vi "VISA_Simple Serial.vi"(0 "VISA resource name":refnum<visa-resource-name>="COM1", 5 "Command":string="*IDN?\\n", 7 "delay before read (ms)":u32=500, 9 "Serial Settings":T1={"baud rate"=9600, "data bits"=8, "parity"=enum."None", "stop bits"=10, "flow control"=0} {"flow control" items=["None"=0, "XON/XOFF"=1, "RTS/CTS"=2, "DTR/DSR"=4]; "stop bits" items=["1.0"=10, "1.5"=15, "2.0"=20]; "data bits" min=5 max=8 step=1; "baud rate" items=["75"=75, "110"=110, "134"=134, "150"=150, "300"=300, "600"=600, "1200"=1200, "1800"=1800, "2400"=2400, "4800"=4800, "7200"=7200, "9600"=9600, "14400"=14400, "19200"=19200, "28800"=28800, "38400"=38400, "56000"=56000, "57600"=57600, "115200"=115200, "128000"=128000, "230400"=230400]}, 11 "error in (no error)":errorcluster) -> (4 "Response":string, 6 "bytes read":u32, 15 "error out":errorcluster)   [LabVIEW 2021, in "Communication.lvlib"]
doc: "<B>Note: This VI is taken from LabVIEW example located at C:\\Program Files (x86)\\National Instruments\\LabVIEW <version>\\examples\\Instrument IO\\Serial\\Simple Serial.vi. More such examples can be found in the same location.</B>\n\nThis example performs a serial port write and a serial port read. The parameters set for the serial port must match the parameters of the connected instrument or device. The VISA Configure Serial Port VI sets the configuration parameters. The front panel displays the controls used to configure the basic parameters, such as baud rate, data bits, and parity. The VI passes the VISA resource name to other VIs that perform operations on that VISA resource. The VISA Write function sends a command to the serial device and the VISA Read function returns data based on the command. The VISA Close function then closes the reference to the serial device. It is important to close the reference; otherwise, further communication through that port might not be possible."
uses:
  Communication.lvlib
  Typedefs/Serial - Settings.ctl
  <vilib>/Instr/_visa.llb/VISA Configure Serial Port (Instr).vi
panel:
  # "Overview: Demonstrates the use of the VISA functions to send a single command to a serial instrument and read a response.\nRequirements: NI-VISA Driver\nInstructions:\n1. Ensure the resource specified by the VISA resource name is a valid serial device.\n2. Enter the serial visa command / query.\n3. Update other configuration required to establish serial communication.\n4. Run the VI."
  # "Note: This VI is taken from LabVIEW example located at C:\\Program Files (x86)\\National Instruments\\LabVIEW <version>\\examples\\Instrument IO\\Serial\\Simple Serial.vi.  More such examples can be found in the same location."
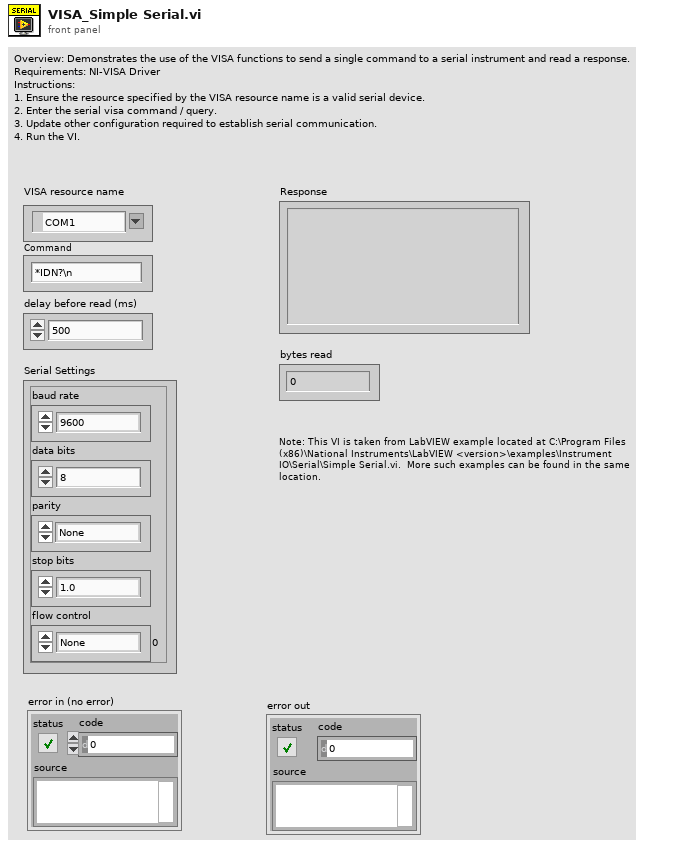
[diagram p1: front panel]
types:
  T1 = typedef "Communication.lvlib/Serial - Settings.ctl" = cluster{"baud rate":u32, "data bits":u16, "parity":enum16{"None", "Odd", "Even", "Mark", "Space"}, "stop bits":u16, "flow control":u16}
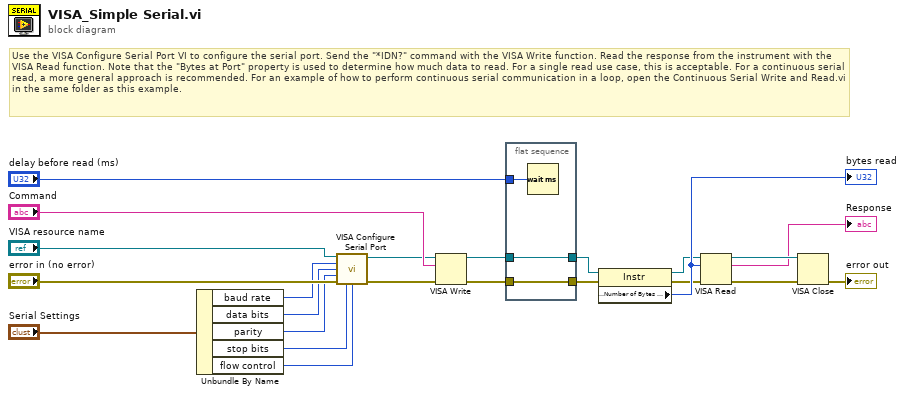
[diagram p0: block diagram]
diagram:
  # "Use the VISA Configure Serial Port VI to configure the serial port. Send the \"*IDN?\" command with the VISA Write function. Read the response from the instrument with the VISA Read function. Note that the \"Bytes at Port\" property is used to determine how much data to read. For a single read use case, this is acceptable. For a continuous serial read, a more general approach is recommended. For an example of how to perform continuous serial communication in a loop, open the Continuous Serial Write and Read.vi in the same folder as this example."
  n1 = Unbundle By Name("Serial Settings") -> ("baud rate"=w9:u32, "data bits"=w8:u16, "parity"=w7:enum16{"None", "Odd", "Even", "Mark", "Space"}, "stop bits"=w6:u16, "flow control"=w5:u16)
  n2 = call-poly "VISA Configure Serial Port"("VISA resource name"="VISA resource name", "baud rate (9600)"=w9, "data bits (8)"=w8, "parity (0:none)"=w7, "error in (no error)"="error in (no error)", "stop bits (10: 1 bit)"=w6, "flow control (0:none)"=w5) -> ("VISA resource name out"=w10:refnum<visa-resource-name>, "error out"=w11:errorcluster)  [unwired: 2 in, 5 out]
  n3 = VISA Write(VISA resource name=w10, write buffer="Command", error in (no error)=w11) -> (VISA resource name out=w19:refnum<visa-resource-name>, error out=w20:errorcluster)  [unwired: 1 out]
  n4 = flat-sequence {
    tunnel: w20 -> [w25]
    tunnel: [w25] -> w4
    tunnel: w19 -> [w24]
    tunnel: [w24] -> w3
    tunnel: "delay before read (ms)" -> [w26]
    frame #0 {
      n5 = Wait (ms)(milliseconds to wait=w26) -> ()  [unwired: 1 out]
    }
  }
  n6 = property class="Instr"(reference=w3, error in=w4) -> (reference out=w2:refnum<visa-resource-name>, error out=w1:errorcluster, "Serial Settings:Number of Bytes at Serial Port"=w16:u32)
  "bytes read" <- w16
  n7 = VISA Read(VISA resource name=w2, byte count=w16, error in (no error)=w1) -> (VISA resource name out=w21:refnum<visa-resource-name>, read buffer=→"Response":string, error out=w22:errorcluster)  [unwired: 1 out]
  n8 = VISA Close(VISA resource name=w21, error in (no error)=w22) -> (error out=→"error out":errorcluster)
